vi "Meter Detection Initialization VI.vi"(8 "error in (no error)":errorcluster, 10 "Custom XML":string, 11 "Device Item Ref in":T1 format="%.0x") -> (0 "error out":errorcluster, 3 "Device Item Ref out":T1 format="%.0x")   [LabVIEW 2011, in "Meter Detection Custom Device.lvlib"]
uses:
  Meter Detection Custom Device.lvlib
  <vilib>/NI Veristand/Custom Device API/Custom Device Item Ref.ctl
  <vilib>/NI Veristand/Custom Device API/Custom Device Channel.ctl
  <vilib>/NI Veristand/Custom Device API/Custom Device Channel Type.ctl
  Shared/Meter Detection Global Variable.vi
  <vilib>/NI Veristand/Custom Device API/Custom Device API.lvlib
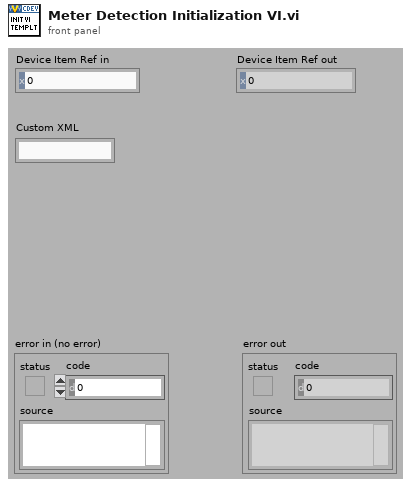
[diagram p1: front panel]
types:
  T1 = typedef "Custom Device API.lvlib/Custom Device Item Ref.ctl" = u64
  T2 = cluster{"Global Rectangle":i32[], "Contours":cluster{"Contour Type":u32, "ROI Type":u32, "Points":i32[]}[]}
  T3 = typedef "Custom Device API.lvlib/Custom Device Channel.ctl" = cluster{"Type":T4, "Units":string, "Default Value":dbl, "Faultable":bool, "Scalable":bool}
  T4 = typedef "Custom Device API.lvlib/Custom Device Channel Type.ctl" = enum16{"Input", "Output"}
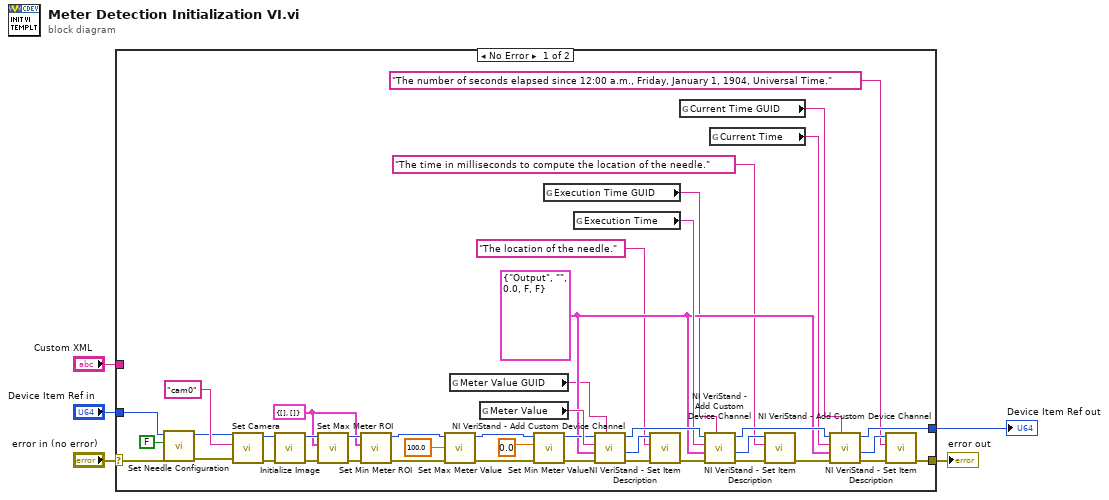
[diagram p0: block diagram]
diagram:
  n1 = case shown="No Error" "error in (no error)" {
    selector: "error in (no error)" -> [w9 w50]
    tunnel: [w15 w50] -> w5
    tunnel: [w30 w49] -> w3
    tunnel: "Device Item Ref in" -> [w6 w49]
    tunnel: "Custom XML" -> [_ _]
    frame No Error {
      w38 = T2 {"Global Rectangle"=[], "Contours"=[]} ("ROI")
      w29 = T3 {"Type"=enum."Output", "Units"="", "Default Value"=0.0, "Faultable"=FALSE, "Scalable"=FALSE} ("Channel")
      n2 = call "Set Needle Configuration.vi"("error in (no error)"=w9, "Needle Configuration in"=FALSE, "Item Ref in"=w6) -> ("error out"=w8:errorcluster, "Item Ref out"=w7:T1)  [unwired: 6 in, 1 out]
      n3 = call "Set Camera.vi"("error in (no error)"=w8, "Camera"="cam0", "Item Ref in"=w7) -> ("error out"=w44:errorcluster, "Item Ref out"=w43:T1)  [unwired: 7 in]
      n4 = call "Initialize Image.vi"("error in (no error)"=w44, "Item Ref in"=w43) -> ("error out"=w42:errorcluster, "Item Ref out"=w41:T1)  [unwired: 8 in]
      n5 = call "Set Max Meter ROI.vi"("error in (no error)"=w42, "ROI"=w38, "Item Ref in"=w41) -> ("error out"=w40:errorcluster, "Item Ref out"=w39:T1)  [unwired: 7 in]
      n6 = call "Set Min Meter ROI.vi"("error in (no error)"=w40, "ROI"=w38, "Item Ref in"=w39) -> ("error out"=w37:errorcluster, "Item Ref out"=w36:T1)  [unwired: 7 in]
      n7 = call "Set Max Meter Value.vi"("error in (no error)"=w37, "Min Gauge Value"=100.0, "Item Ref in"=w36) -> ("error out"=w35:errorcluster, "Item Ref out"=w34:T1)  [unwired: 7 in]
      n8 = global read "Meter Detection Global Variable.vi" "Meter Value GUID"() -> (w27:string)
      n9 = global read "Meter Detection Global Variable.vi" "Meter Value"() -> (w48:string)
      n10 = call "Set Min Meter Value.vi"("error in (no error)"=w35, "Min Gauge Value"=0.0, "Item Ref in"=w34) -> ("error out"=w33:errorcluster, "Item Ref out"=w32:T1)  [unwired: 7 in]
      n11 = global read "Meter Detection Global Variable.vi" "Execution Time GUID"() -> (w26:string)
      n12 = global read "Meter Detection Global Variable.vi" "Execution Time"() -> (w46:string)
      n13 = call <vilib>:"NI VeriStand - Add Custom Device Channel.vi"("GUID (Default Channel)"=w27, "error in (no error)"=w33, "Channel"=w29, "Channel Name"=w48, "Parent Ref in"=w32) -> ("error out"=w24:errorcluster, "Channel Ref"=w23:T1, "Parent Ref out"=w47:T1)  [unwired: 3 in, 1 out]
      n14 = call <vilib>:"NI VeriStand - Set Item Description.vi"("error in (no error)"=w24, "Description"="The location of the needle.", "Item Ref in"=w23) -> ("error out"=w22:errorcluster)  [unwired: 6 in, 2 out]
      n15 = global read "Meter Detection Global Variable.vi" "Current Time GUID"() -> (w25:string)
      n16 = call <vilib>:"NI VeriStand - Add Custom Device Channel.vi"("GUID (Default Channel)"=w26, "error in (no error)"=w22, "Channel"=w29, "Channel Name"=w46, "Parent Ref in"=w47) -> ("error out"=w19:errorcluster, "Channel Ref"=w20:T1, "Parent Ref out"=w31:T1)  [unwired: 3 in, 1 out]
      n17 = global read "Meter Detection Global Variable.vi" "Current Time"() -> (w28:string)
      n18 = call <vilib>:"NI VeriStand - Set Item Description.vi"("error in (no error)"=w19, "Description"="The time in milliseconds to compute the location of the needle.", "Item Ref in"=w20) -> ("error out"=w18:errorcluster)  [unwired: 6 in, 2 out]
      n19 = call <vilib>:"NI VeriStand - Add Custom Device Channel.vi"("GUID (Default Channel)"=w25, "error in (no error)"=w18, "Channel"=w29, "Channel Name"=w28, "Parent Ref in"=w31) -> ("error out"=w16:errorcluster, "Channel Ref"=w14:T1, "Parent Ref out"=w30:T1)  [unwired: 3 in, 1 out]
      n20 = call <vilib>:"NI VeriStand - Set Item Description.vi"("error in (no error)"=w16, "Description"="The number of seconds elapsed since 12:00 a.m., Friday, January 1, 1904, Universal Time.", "Item Ref in"=w14) -> ("error out"=w15:errorcluster)  [unwired: 6 in, 2 out]
    }
    frame Error {
    }
  }
  "error out" <- w5
  "Device Item Ref out" <- w3
